vi "Revert.vi"(8 "error in (no error)":errorcluster, 11 "Git Updater Module in":refnum<class "Git Updater Module.lvclass">) -> (0 "error out":errorcluster, 3 "Git Updater Module out":refnum<class "Git Updater Module.lvclass">)   [LabVIEW 2020, in "VolatusGUI.lvlib" / "Git Updater Module.lvclass"]
uses:
  Git Updater Module.lvclass
  Git Updater Module.lvclass/Git Updater Module.ctl
  <vilib>/Hampel Software Engineering/Git API/Git API/GIT-api.lvclass
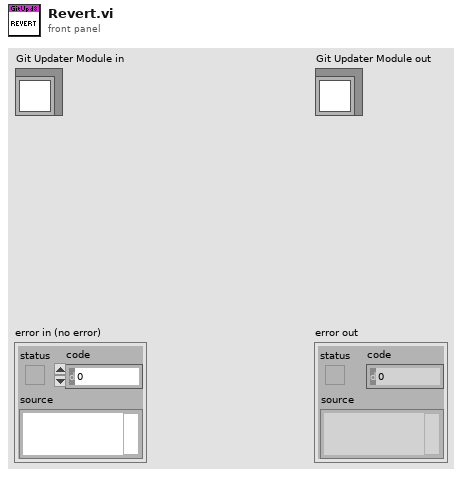
[diagram p1: front panel]
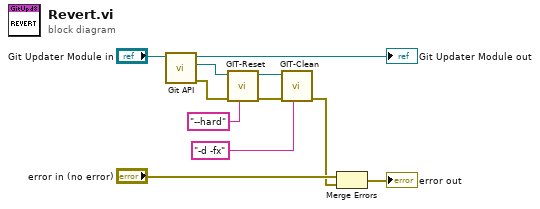
[diagram p0: block diagram]
diagram:
  n1 = call "Git API.vi"("Git Updater Module in"="Git Updater Module in") -> ("error out"=w7:errorcluster, "git-api"=w8:refnum<class "GIT-api.lvclass">, "Git Updater Module out"=→"Git Updater Module out":refnum<class "Git Updater Module.lvclass">)  [unwired: 8 in]
  n2 = call <vilib>:"GIT-Reset.vi"("param"="--hard", "error in"=w7, "git-api in"=w8) -> ("error out"=w4:errorcluster, "git-api out"=w5:refnum<class "GIT-api.lvclass">)  [unwired: 6 in, 1 out]
  n3 = call <vilib>:"GIT-Clean.vi"("param"="-d -fx", "error in"=w4, "Git-API in"=w5) -> ("error out"=w1:errorcluster)  [unwired: 6 in, 2 out]
  n4 = Merge Errors("error in (no error)", w1) -> (→"error out":errorcluster)
